vi "Clean names.vi"(11 "Name with extension":string) -> (3 "Name without extension":string)   [LabVIEW 2020, in "Test Tree.lvclass"]
uses:
  Test Tree.lvclass
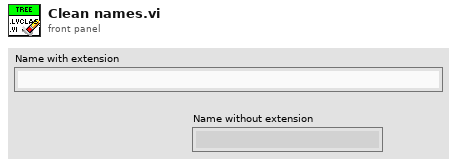
[diagram p1: front panel]
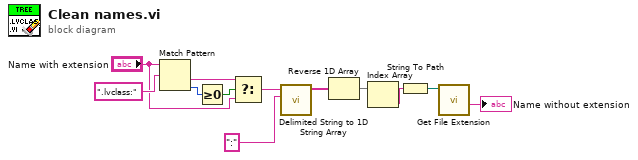
[diagram p0: block diagram]
diagram:
  n1 = Match Pattern(string="Name with extension", regular expression=".lvclass:") -> (after substring=w7:string, offset past match=w10:i32)  [unwired: 1 in, 2 out]
  n2 = Greater Or Equal To 0?(x=w10) -> (x >= 0?=w9:bool)
  n3 = Select(t=w7, s=w9, f="Name with extension") -> (s? t:f=w5:string)
  n4 = call <vilib>:"Delimited String to 1D String Array.vi"("delimiter"=":" ("search string"), "delimited string"=w5) -> ("string array"=w3:string[])  [unwired: 9 in]
  n5 = Reverse 1D Array(array=w3) -> (reversed array=w2:string[])
  n6 = Index Array(array=w2) -> (element=w1:string)  [unwired: 1 in]
  n7 = String To Path(string=w1) -> (path=w8:path)
  n8 = call <vilib>:"Get File Extension.vi"("file"=w8) -> ("filename without extension"=→"Name without extension":string)  [unwired: 6 in, 4 out]
